vi "Write.vi"(0 "Timeout mS (-1)":i32, 2 "element":T1, 3 "Close? (F)":bool) -> (1 "Timed Out?":bool, 4 "Closed?":bool, 6 "channel":T2)   [LabVIEW 2020, in "Flex.lvlib"]
doc: "Writes a value to a Tag channel."
uses:
  Flex.lvlib
  ))Channel.ctl
  Element.ctl
  ChannelOp.ctl
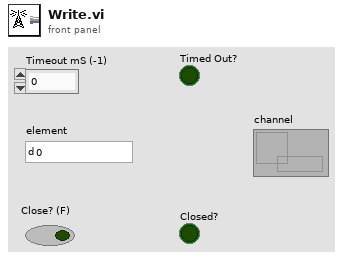
[diagram p1: front panel]
types:
  T1 = typedef "Flex.lvlib/Element.ctl" = dbl
  T2 = typedef "Flex.lvlib/))Channel.ctl" = refnum<queue>
  T3 = typedef "Flex.lvlib/ChannelOp.ctl" = enum16{"Get Refs", "Init", "Close", "Probe", "New Queue", "Remove Queue"}
  T4 = typedef "Flex.lvlib/Channel Data.ctl" = cluster{"Element":refnum<data-value>, "Queue Refs":refnum<data-value>, "Update":refnum<k4>}
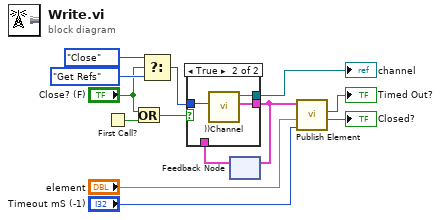
[diagram p0: block diagram]
diagram:
  n1 = First Call?() -> (First Call?: T/F=w9:bool)
  n2 = Or(x="Close? (F)", y=w9) -> (x .or. y?=w10:bool)
  n3 = Select(t=ChannelOp."Close" ("channelOp"), s="Close? (F)", f=ChannelOp."Get Refs" ("channelOp")) -> (s? t:f=w8:T3)
  n4 = feedback #1() -> (w13:T4)  [unwired: 1 in]
  n5 = case shown="True" w10 {
    tunnel: w8 -> [_ w17]
    tunnel: w13 -> [w14 _]
    tunnel: [w14 w15] -> w6
    tunnel: [_ w16] -> w1
    frame False {
    }
    frame True {
      n6 = call "))Channel.vi"("channelOp"=w17) -> ("Channel Data"=w15:T4, "channel out"=w16:T2)  [unwired: 7 in, 2 out]
    }
  }
  "channel" <- w1
  n7 = feedback-in #1(w6) -> ()
  n8 = call "Publish Element.vi"("Timeout mS (-1)"="Timeout mS (-1)", "element"="element", "Channel Data In"=w6) -> ("Closed"=→"Closed?":bool, "Timeout"=→"Timed Out?":bool)  [unwired: 7 in]
